vi "I2C Open.vi"(8 "Error In":errorcluster, 10 "I2C Channel (0)":u8, 11 "LINX Device Config":T1) -> (0 "Error Out":errorcluster, 3 "LINX Device Config":T1)   [LabVIEW 2020, in "Device.lvlib"]
doc: "Open the selected I2C channel and join bus as I2C master."
uses:
  Device.lvlib
  Type Defs/Error Type.ctl
  LMH-LINX.lvlib
  Type Defs/Interface.ctl
  Type Defs/Channels.ctl
  Type Defs/TCP Config.ctl
  Type Defs/LINX Device Config.ctl
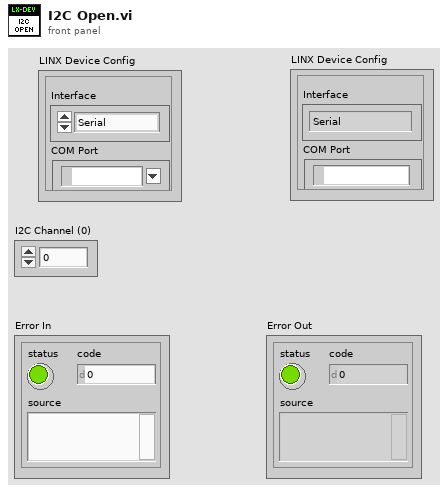
[diagram p1: front panel]
types:
  T1 = typedef "Device.lvlib/LINX Device Config.ctl" = cluster{"Interface":T2, "COM Port":refnum<visa-resource-name>, "TCP Configuration":T3, "Device Family":u8, "Device ID":u8, "Device Name":string, "TCP Ref":refnum<k5>, "Channels":T4}
  T2 = typedef "LMH-LINX.lvlib/Interface.ctl" = enum16{"Serial", "TCP"}
  T3 = typedef "Device.lvlib/TCP Config.ctl" = cluster{"IP Address":string, "Port":u16}
  T4 = typedef "LMH-LINX.lvlib/Channels.ctl" = cluster{"DI":u8[], "DO":u8[], "AI":u8[], "AO":u8[], "PWM":u8[], "QE":u8[], "UART":u8[], "I2C 2":u8[], "SPI":u8[], "CAN":u8[], "Servo":u8[], "AI Ref (V)":dbl, "AI Resolution (Bits)":u8, "AO Ref (V)":dbl, "AO Resolution (Bits)":u8}
  T5 = typedef "LMH-LINX.lvlib/Error Type.ctl" = enum16{"Unknown", "Timeout", "Corrupt Return Packet", "Unable To Connect", "Command Not Supported", "Channel DNE", "Invalid COM Config", "Firmware Version Mismatch", "myRIO Support", "CMD Specific Error", "Local IO Not Supported"}
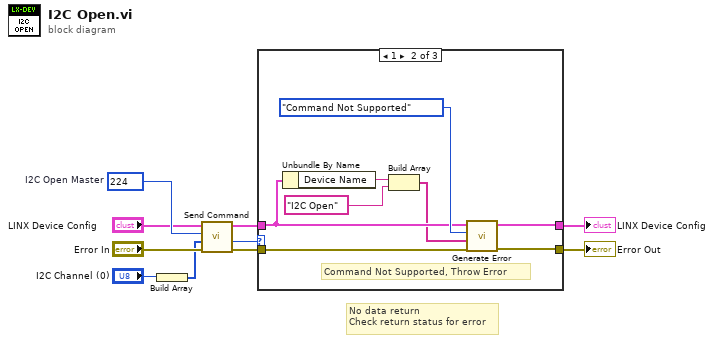
[diagram p0: block diagram]
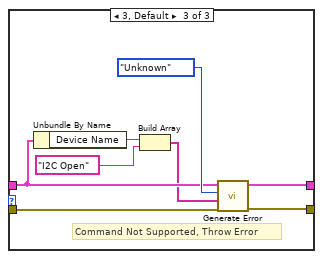
[diagram p3: hidden frame]
diagram:
  w9 = u16 224  # I2C Open Master
  # "No data return\nCheck return status for error"
  n1 = Build Array("I2C Channel (0)") -> (w2:u8[])
  n2 = call "Send Command.vi"("Error In"="Error In", "ARGS"=w2, "CMD"=w9, "LINX Device Config"="LINX Device Config") -> ("Error Out"=w4:errorcluster, "Status"=w1:u8, "LINX Device Config"=w6:T1)  [unwired: 4 in, 1 out]
  n3 = case shown="1" w1 {
    tunnel: [w12 w18 w26] -> w7
    tunnel: w6 -> [w12 w14 w22]
    tunnel: [w11 w19 w27] -> w5
    tunnel: w4 -> [w11 w20 w28]
    frame 0 {
      # "Status OK, Process Data"
    }
    frame 1 {
      # "Command Not Supported, Throw Error"
      n4 = Unbundle By Name(w14) -> ("Device Name"=w16:string)
      n5 = Build Array(w16, "I2C Open") -> (w13:string[])
      n6 = call "Generate Error.vi"("Error In"=w20, "Arguments"=w13, "Error Type"=Error_Type."Command Not Supported", "LINX Device Config"=w14) -> ("Error Out"=w19:errorcluster, "Dup LINX Device Config"=w18:T1)  [unwired: 6 in]
    }
    frame 3, Default {
      # "Command Not Supported, Throw Error"
      n7 = Unbundle By Name(w22) -> ("Device Name"=w24:string)
      n8 = Build Array(w24, "I2C Open") -> (w21:string[])
      n9 = call "Generate Error.vi"("Error In"=w28, "Arguments"=w21, "Error Type"=Error_Type."Unknown", "LINX Device Config"=w22) -> ("Error Out"=w27:errorcluster, "Dup LINX Device Config"=w26:T1)  [unwired: 6 in]
    }
  }
  "Error Out" <- w5
  "LINX Device Config" <- w7
